vi "Move.vi"(8 "error in (no error)":errorcluster, 10 "degrees To move":dbl, 11 "Motor in":refnum<class "Motor.lvclass">) -> (0 "error out":errorcluster, 3 "Motor out":refnum<class "Motor.lvclass">)   [LabVIEW 2019, in "Motor.lvclass"]
uses:
  Motor.lvclass
  Motor.lvclass/Motor.ctl
  Motor Serial class/Serial.lvclass
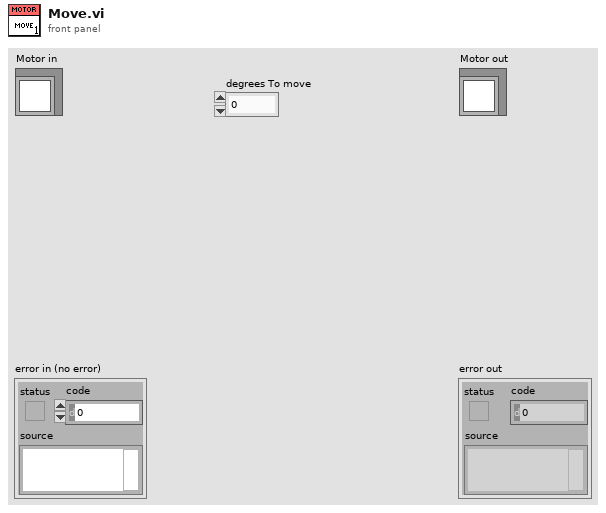
[diagram p1: front panel]
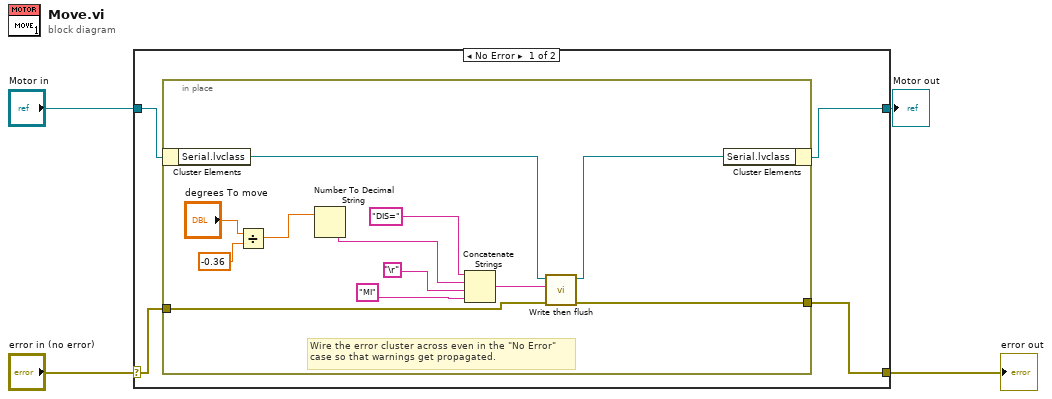
[diagram p0: block diagram]
diagram:
  n1 = case shown="No Error" "error in (no error)" {
    selector: "error in (no error)" -> [w6 w22]
    tunnel: [w5 w22] -> w3
    tunnel: [w7 w21] -> w1
    tunnel: "Motor in" -> [w8 w21]
    frame No Error {
      n2 = in-place {
        in-place-border: w6 -> [w11]
        in-place-border: [w9] -> w5
        # "Wire the error cluster across even in the \"No Error\"\ncase so that warnings get propagated."
        n3 = in-place-cluster #1(w8) -> ("Serial.lvclass"=w13:refnum<class "Serial.lvclass">)
        n4 = Divide(x="degrees To move", y=-0.36) -> (x/y=w17:dbl)
        n5 = Number To Decimal String(number=w17) -> (decimal integer string=w15:string)  [unwired: 1 in]
        n6 = Concatenate Strings("DIS=" ("string"), w15, "\r", "MI" ("string")) -> (w12:string)
        n7 = call "Write then flush.vi"("error in (no error)"=w11, "TX Data"=w12, "Motor_Serial in"=w13) -> ("error out"=w9:errorcluster, "Motor_Serial out"=w10:refnum<class "Serial.lvclass">)  [unwired: 7 in]
        n8 = in-place-cluster #1("Serial.lvclass"=w10) -> (w7:refnum<class "Motor.lvclass">)
      }
    }
    frame Error {
    }
  }
  "error out" <- w3
  "Motor out" <- w1
